vi "PXI6120_tio.vi"() -> ()   [LabVIEW 2017]
doc: "Use this template to build a producer/consumer design pattern with events to produce queue items. Use this design pattern instead of the User Interface Event Handler pattern for user interfaces when you want to execute code asynchronously in response to an event without slowing the user interface responsiveness."
uses:
  controls/FS_PXI6602TIO.ctl
  <vilib>/DAQmx/read.llb/DAQmx Read (Counter U32 1Chan 1Samp).vi
  <vilib>/DAQmx/create/channels.llb/DAQmx Create Channel (CO-Pulse Generation-Frequency).vi
  <vilib>/DAQmx/configure/timing.llb/DAQmx Timing (Implicit).vi
  <vilib>/DAQmx/create/channels.llb/DAQmx Create Channel (CI-Count Edges).vi
  <vilib>/DAQmx/miscellaneous.llb/DAQmx Fill In Error Info.vi
  <resource>/objmgr/daqmx.rc
panel:
  in  "Counter":bool
  in  "Active Edge":i32(ring)=10171 items=["Rising"=10280, "Falling"=10171]
  out "Count":u32
  in  "Input Terminal":tag="/Dev2/PFI3"
  in  "Counter in":tag="Dev2/ctr1"
  in  "Loop Time (ms)":u32=10
  in  "Pulse":bool
  out "Actual Duty Cycle":dbl
  out "Actual Frequency":dbl
  in  "Duty Cycle":dbl=0.5 format="%.6f"
  in  "Frequency":dbl=1.0 format="%.6f"
  in  "Output Terminal":tag
  in  "Counter out":tag="Dev2/ctr0"
  # "PXI-6120计数器信号输出/输出"
  # "Channel Settings"
  # "Channel Settings"
  # "Acquired Data"
  # "Timing Settings"
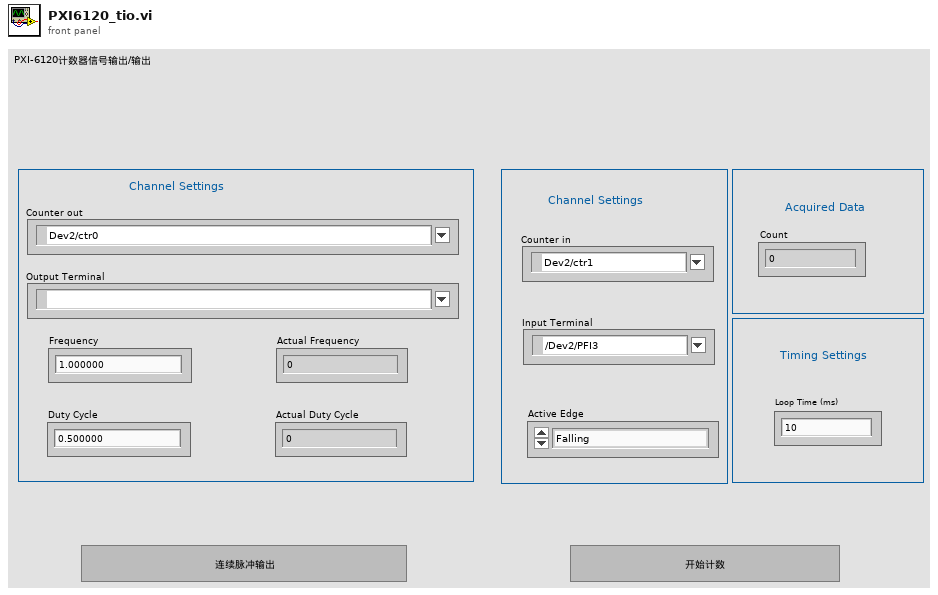
[diagram p1: front panel]
types:
  T1 = typedef "FS_PXI6602TIO.ctl" = enum16{"Initialize", "Start TO", "Start Counter", "Read data", "Stop TO", "Stop Counter", "Idel"}
  T2 = cluster{"Pulse":refnum<k21>, "Counter":refnum<k21>}
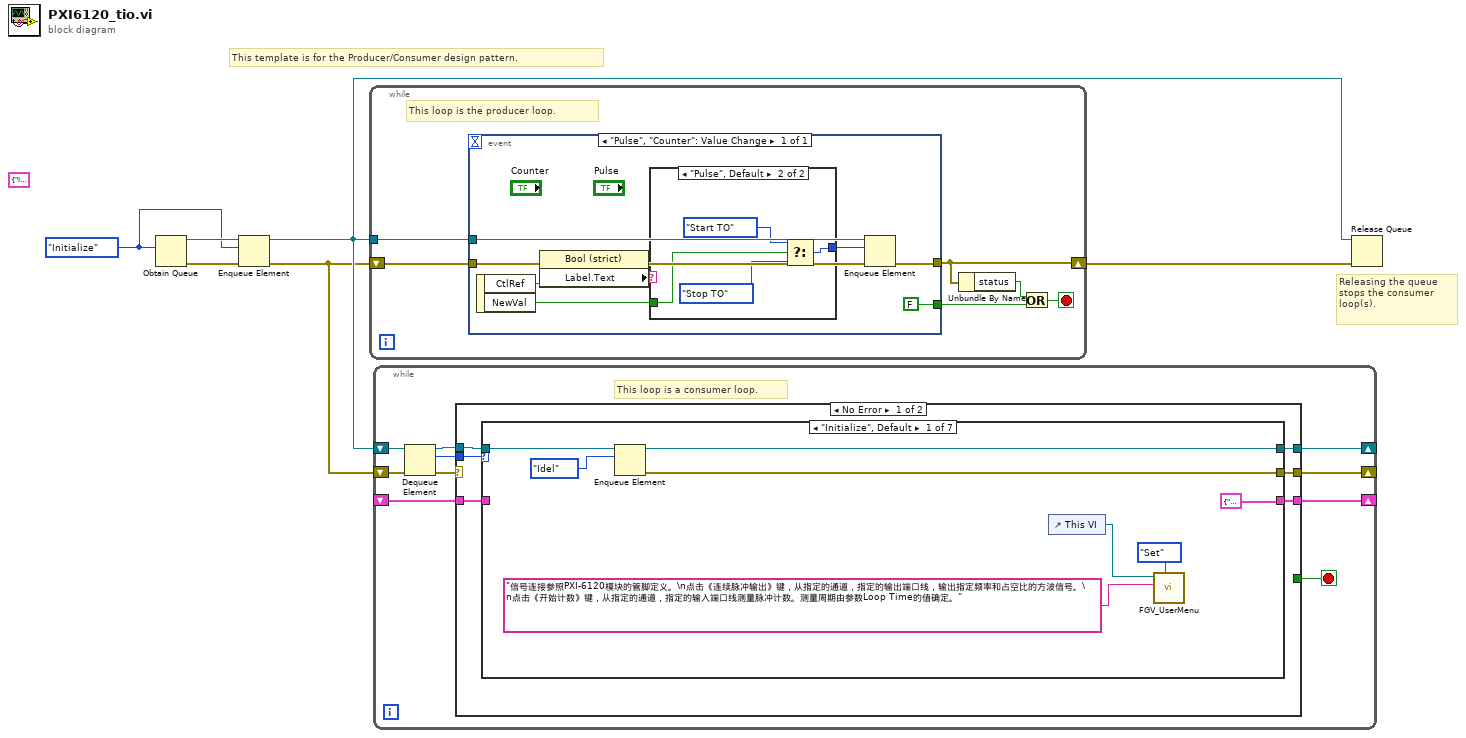
[diagram p0: block diagram]
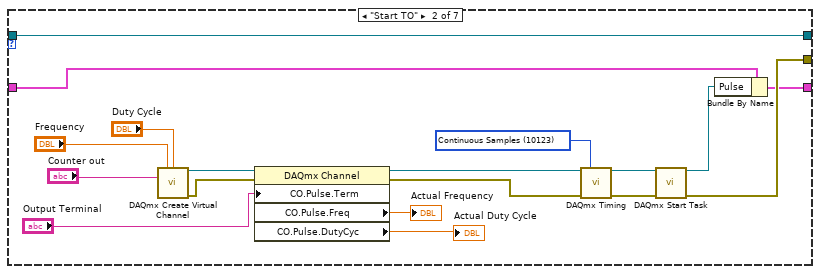
[diagram p2: hidden frame]
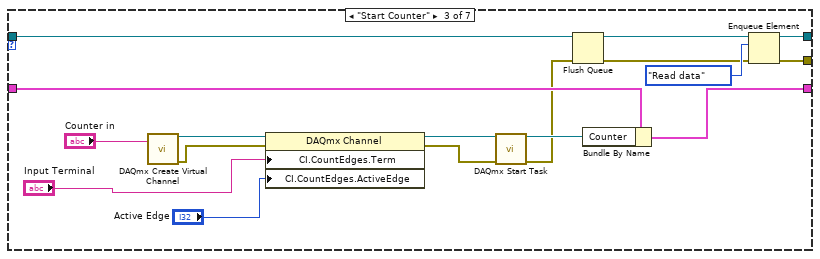
[diagram p3: hidden frame]
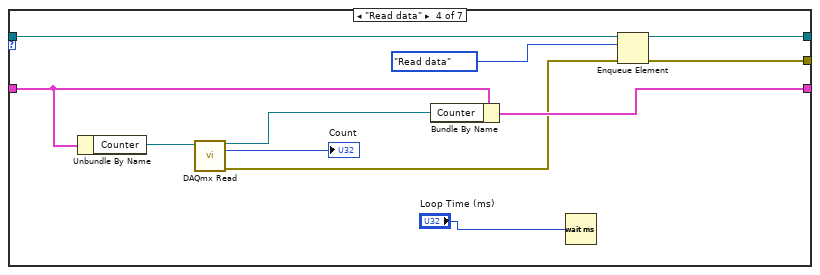
[diagram p4: hidden frame]
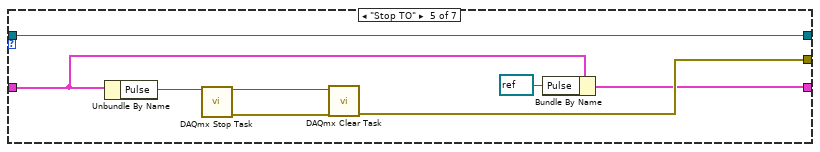
[diagram p5: hidden frame]
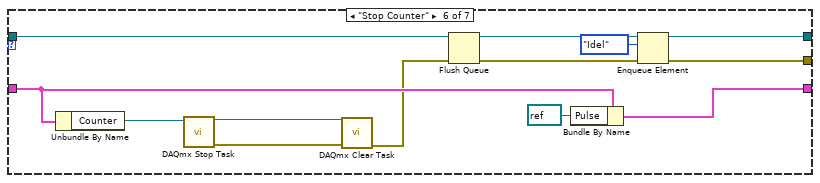
[diagram p6: hidden frame]
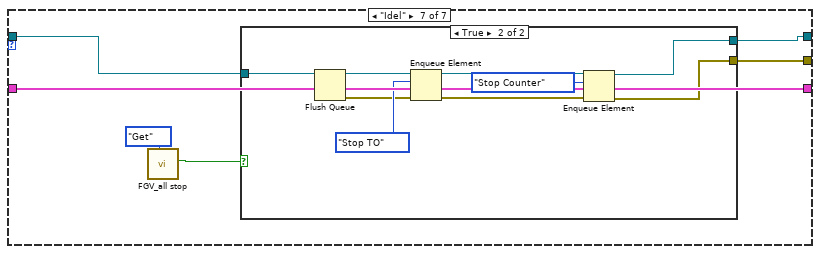
[diagram p7: hidden frame]
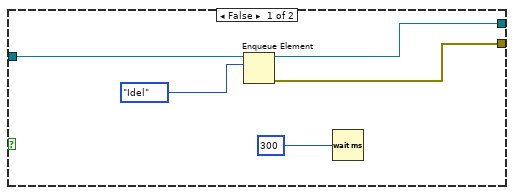
[diagram p8: hidden frame]
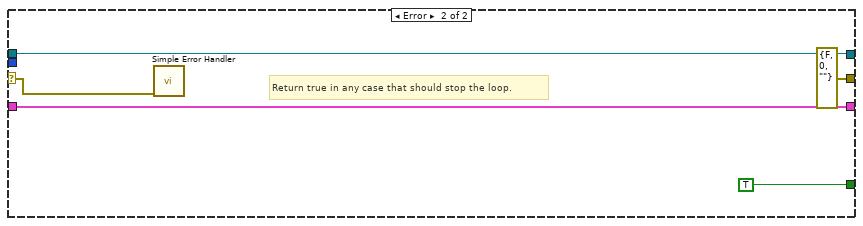
[diagram p9: hidden frame]
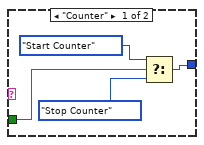
[diagram p10: hidden frame]
diagram:
  (unwired) cluster{"Command":T1, "Data":variant} {"Command"=enum."Initialize", "Data"=variant}
  w2 = FS_PXI6602TIO."Initialize"
  # "Releasing the queue stops the consumer loop(s)."
  # "This template is for the Producer/Consumer design pattern."
  n1 = Obtain Queue(element data type=w2) -> (queue out=w5:refnum<queue>, error out=w3:errorcluster)  [unwired: 4 in, 1 out]
  n2 = Enqueue Element(queue=w5, element=w2, error in (no error)=w3) -> (queue out=w4:refnum<queue>, error out=w1:errorcluster)  [unwired: 1 in, 1 out]
  n3 = while {
    shift-right: [w8] -> w6
    shift-left: w1 -> [w11]
    tunnel: w4 -> [w12]
    stop <- w9 stop-if-true
    # "This loop is the producer loop."
    n4 = event shown="[0] \"Pulse\", \"Counter\": Value Change" {
      selector: _ -> [_]
      dyn-events: _ -> [_]
      timeout: _ -> [_]
      tunnel: w12 -> [w19]
      tunnel: w11 -> [w21]
      tunnel: [w20] -> w8
      tunnel: [FALSE] -> w10
      event "Pulse", "Counter": Value Change {
        n5 = event-data() -> ("CtlRef"=w16:refnum<vi>, "NewVal"=w14:bool)  [unwired: 1 in]
        n6 = property class="Bool (strict)"(reference=w16, error in=w21) -> (error out=w17:errorcluster, "Label.Text"=w15:string)  [unwired: 1 out]
        n7 = case shown="\"Pulse\", Default" w15 {
          tunnel: w14 -> [w25 w29]
          tunnel: [w22 w26] -> w13
          frame "Counter" {
            n8 = Select(t=FS_PXI6602TIO."Start Counter", s=w25, f=FS_PXI6602TIO."Stop Counter") -> (s? t:f=w22:T1)
          }
          frame "Pulse", Default {
            n9 = Select(t=FS_PXI6602TIO."Start TO", s=w29, f=FS_PXI6602TIO."Stop TO") -> (s? t:f=w26:T1)
          }
        }
        n10 = Enqueue Element(queue=w19, element=w13, error in (no error)=w17) -> (error out=w20:errorcluster)  [unwired: 1 in, 2 out]
      }
    }
    n11 = Unbundle By Name(w8) -> ("status"=w7:bool)
    n12 = Or(x=w7, y=w10) -> (x .or. y?=w9:bool)
  }
  n13 = while {
    shift-right: [w33] -> _
    shift-left: w1 -> [w35]
    shift-right: [w32] -> _
    shift-left: _ -> [w31]
    shift-right: [w30] -> _
    shift-left: w4 -> [w39]
    stop <- w36 stop-if-true
    # "This loop is a consumer loop."
    n14 = Dequeue Element(queue=w39, error in (no error)=w35) -> (queue out=w34:refnum<queue>, element=w37:T1, error out=w38:errorcluster)  [unwired: 1 in, 1 out]
    n15 = case shown="No Error" w38 {
      selector: w38 -> [_ w143]
      tunnel: w37 -> [w45 _]
      tunnel: [_ TRUE] -> w36
      tunnel: w34 -> [w44 w144]
      tunnel: [w43 errorcluster {"status"=FALSE, "code"=0, "source"=""} ("error out")] -> w33
      tunnel: [w42 w142] -> w32
      tunnel: w31 -> [w41 w142]
      tunnel: [w40 w144] -> w30
      frame No Error {
        n16 = case shown="\"Initialize\", Default" w45 {
          tunnel: w44 -> [w53 w54 w78 w93 w100 w114 w123]
          tunnel: [w51 w58 w76 w90 w104 w109 w122] -> w43
          tunnel: [T2 {"Pulse"="", "Counter"=""} w56 w79 w95 w101 w115 w126] -> w42
          tunnel: w41 -> [_ w55 w81 w97 w103 w117 w126]
          tunnel: [w49 w54 w77 w92 w100 w111 w121] -> w40
          frame "Initialize", Default {
            n17 = Enqueue Element(queue=w53, element=FS_PXI6602TIO."Idel") -> (queue out=w49:refnum<queue>, error out=w51:errorcluster)  [unwired: 2 in, 1 out]
            n18 = control-ref of="This VI"() -> (w47:refnum<vi>)
            n19 = call "FGV_UserMenu.vi"("Command"=enum16{"Initialize", "Set", "Get"}."Set", "Use Info"="信号连接参照PXI-6120模块的管脚定义。\n点击《连续脉冲输出》键，从指定的通道，指定的输出端口线，输出指定频率和占空比的方波信号。\n点击《开始计数》键，从指定的通道，指定的输入端口线测量脉冲计数。测量周期由参数Loop Time的值确定。", "VI Refnum"=w47) -> ()  [unwired: 8 in, 1 out]
          }
          frame "Start TO" {
            w61 = 10123 items=["Finite Samples"=10178, "Continuous Samples"=10123, "Hardware Timed Single Point"=12522] ("sample mode")
            n20 = call-poly <vilib>:"DAQmx Create Virtual Channel.vi"("frequency"="Frequency", "duty cycle"="Duty Cycle", "counter"="Counter out") -> ("task out"=w67:refnum<k21>, "error out"=w68:errorcluster)  [unwired: 11 in]
            n21 = property class="DAQmx Channel"(reference=w67, error in=w68, "CO.Pulse.Term"="Output Terminal") -> (reference out=w63:refnum<k21>, error out=w62:errorcluster, "CO.Pulse.Freq"=→"Actual Frequency":dbl, "CO.Pulse.DutyCyc"=→"Actual Duty Cycle":dbl)
            n22 = call-poly <vilib>:"DAQmx Timing.vi"("task/channels in"=w63, "sample mode"=w61, "error in"=w62) -> ("task out"=w60:refnum<k21>, "error out"=w59:errorcluster)  [unwired: 11 in]
            n23 = call <vilib>:"DAQmx Start Task.vi"("task/channels in"=w60, "error in"=w59) -> ("task out"=w57:refnum<k21>, "error out"=w58:errorcluster)  [unwired: 12 in]
            n24 = Bundle By Name(cluster=w55, "Pulse"=w57) -> (w56:T2)
          }
          frame "Start Counter" {
            n25 = call-poly <vilib>:"DAQmx Create Virtual Channel.vi"("counter"="Counter in") -> ("task out"=w87:refnum<k21>, "error out"=w85:errorcluster)  [unwired: 13 in]
            n26 = property class="DAQmx Channel"(reference=w87, error in=w85, "CI.CountEdges.Term"="Input Terminal", "CI.CountEdges.ActiveEdge"="Active Edge") -> (reference out=w83:refnum<k21>, error out=w82:errorcluster)
            n27 = call <vilib>:"DAQmx Start Task.vi"("task/channels in"=w83, "error in"=w82) -> ("task out"=w80:refnum<k21>, "error out"=w73:errorcluster)  [unwired: 12 in]
            n28 = Flush Queue(queue=w78, error in (no error)=w73) -> (queue out=w74:refnum<queue>, error out=w72:errorcluster)  [unwired: 1 out]
            n29 = Bundle By Name(cluster=w81, "Counter"=w80) -> (w79:T2)
            n30 = Enqueue Element(queue=w74, element=FS_PXI6602TIO."Read data", error in (no error)=w72) -> (queue out=w77:refnum<queue>, error out=w76:errorcluster)  [unwired: 1 in, 1 out]
          }
          frame "Read data" {
            n31 = Unbundle By Name(w97) -> ("Counter"=w99:refnum<k21>)
            n32 = call-poly <vilib>:"DAQmx Read.vi"("task/channels in"=w99) -> ("task out"=w96:refnum<k21>, "data"=→"Count":u32, "error out"=w91:errorcluster)  [unwired: 12 in]
            n33 = Bundle By Name(cluster=w97, "Counter"=w96) -> (w95:T2)
            n34 = Wait (ms)(milliseconds to wait="Loop Time (ms)") -> ()  [unwired: 1 out]
            n35 = Enqueue Element(queue=w93, element=FS_PXI6602TIO."Read data", error in (no error)=w91) -> (queue out=w92:refnum<queue>, error out=w90:errorcluster)  [unwired: 1 in, 1 out]
          }
          frame "Stop TO" {
            n36 = Unbundle By Name(w103) -> ("Pulse"=w107:refnum<k21>)
            n37 = call <vilib>:"DAQmx Stop Task.vi"("task/channels in"=w107) -> ("task out"=w106:refnum<k21>, "error out"=w105:errorcluster)  [unwired: 13 in]
            n38 = call <vilib>:"DAQmx Clear Task.vi"("task in"=w106, "error in"=w105) -> ("error out"=w104:errorcluster)  [unwired: 13 in]
            n39 = Bundle By Name(cluster=w103, "Pulse"=refnum<k21> refnum) -> (w101:T2)
          }
          frame "Stop Counter" {
            n40 = Unbundle By Name(w117) -> ("Counter"=w120:refnum<k21>)
            n41 = call <vilib>:"DAQmx Stop Task.vi"("task/channels in"=w120) -> ("task out"=w118:refnum<k21>, "error out"=w119:errorcluster)  [unwired: 13 in]
            n42 = call <vilib>:"DAQmx Clear Task.vi"("task in"=w118, "error in"=w119) -> ("error out"=w112:errorcluster)  [unwired: 13 in]
            n43 = Flush Queue(queue=w114, error in (no error)=w112) -> (queue out=w113:refnum<queue>, error out=w110:errorcluster)  [unwired: 1 out]
            n44 = Bundle By Name(cluster=w117, "Pulse"=refnum<k21> refnum) -> (w115:T2)
            n45 = Enqueue Element(queue=w113, element=FS_PXI6602TIO."Idel", error in (no error)=w110) -> (queue out=w111:refnum<queue>, error out=w109:errorcluster)  [unwired: 1 in, 1 out]
          }
          frame "Idel" {
            n46 = call "FGV_all stop.vi"("Enum"=enum16{"Set", "Get"}."Get") -> ("All Stop?"=w124:bool)  [unwired: 10 in]
            n47 = case shown="True" w124 {
              tunnel: w123 -> [w131 w140]
              tunnel: [w129 w135] -> w122
              tunnel: [w130 w134] -> w121
              frame False {
                n48 = Enqueue Element(queue=w131, element=FS_PXI6602TIO."Idel") -> (queue out=w130:refnum<queue>, error out=w129:errorcluster)  [unwired: 2 in, 1 out]
                n49 = Wait (ms)(milliseconds to wait=300) -> ()  [unwired: 1 out]
              }
              frame True {
                n50 = Flush Queue(queue=w140) -> (queue out=w133:refnum<queue>, error out=w132:errorcluster)  [unwired: 1 in, 1 out]
                n51 = Enqueue Element(queue=w133, element=FS_PXI6602TIO."Stop TO", error in (no error)=w132) -> (queue out=w138:refnum<queue>, error out=w137:errorcluster)  [unwired: 1 in, 1 out]
                n52 = Enqueue Element(queue=w138, element=FS_PXI6602TIO."Stop Counter", error in (no error)=w137) -> (queue out=w134:refnum<queue>, error out=w135:errorcluster)  [unwired: 1 in, 1 out]
              }
            }
          }
        }
      }
      frame Error {
        # "Return true in any case that should stop the loop."
        n53 = call <vilib>:"Simple Error Handler.vi"("error in (no error)"=w143) -> ()  [unwired: 4 in, 5 out]
      }
    }
  }
  n54 = Release Queue(queue=w4, error in (no error)=w6) -> ()  [unwired: 1 in, 3 out]
